vi "Read Test Parameters.vi"(8 "error in":errorcluster) -> (0 "error out":errorcluster, 1 "fbf_2 Pass Criteria":i32=3, 2 "fbf_1 Pass Criteria":i32=10, 3 "Array of tests":T1[](array[typedef]) {"Measurement Res." format="%.0f MHz"; "Blocking Signal" format="%#_gdBm"; "Wanted Signal" format="%#_gdBm"; "Upper Frequency" format="%.0f MHz"; "Lower Frequency" format="%.0f MHz"})   [LabVIEW 2013]
uses:
  Master Test Parameters.ctl
  <vilib>/Utility/config.llb/Config Data RefNum.ctl
  Globals/Blocking Performance Test Application Globals.vi
  <vilib>/Utility/config.llb/Read Key (Double).vi
  Globals/Test Criteria Global.vi
  <vilib>/Utility/config.llb/Read Key (U32).vi
  <vilib>/Utility/config.llb/Read Key (I32).vi
  <vilib>/Utility/config.llb/NI_LVConfig.lvlib
panel:
  out "Sections":i32
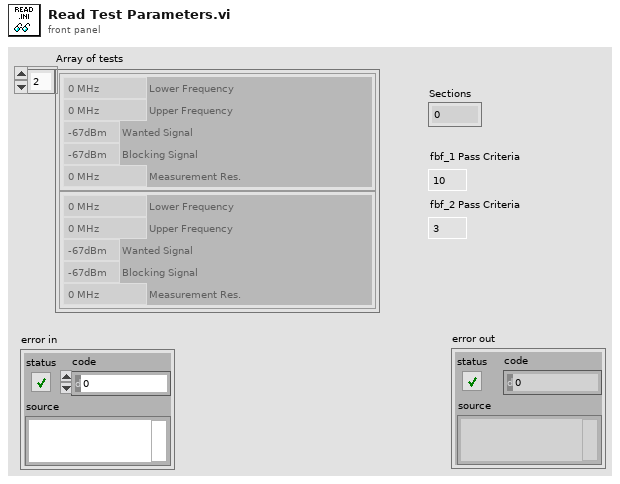
[diagram p1: front panel]
types:
  T1 = typedef "Master Test Parameters.ctl" = cluster{"Lower Frequency":u32, "Upper Frequency":u32, "Wanted Signal":dbl, "Blocking Signal":dbl, "Measurement Res.":u32}
  T2 = typedef "NI_LVConfig.lvlib/Config Data RefNum.ctl" = refnum<k1>
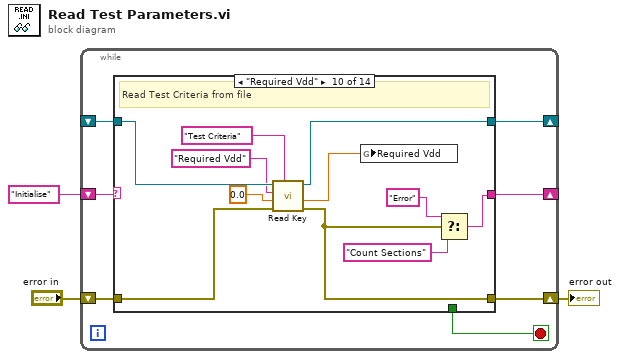
[diagram p0: block diagram]
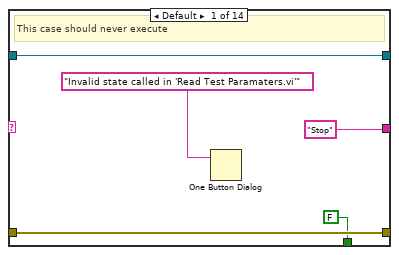
[diagram p2: hidden frame]
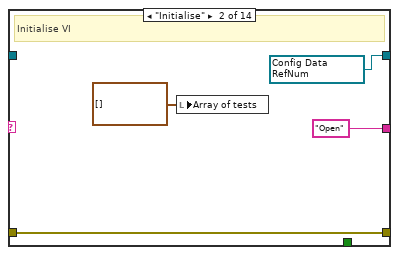
[diagram p3: hidden frame]
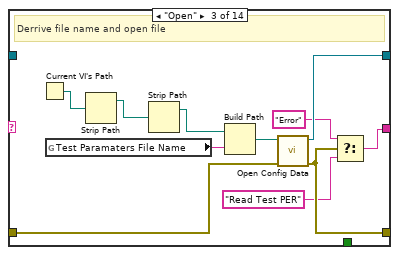
[diagram p4: hidden frame]
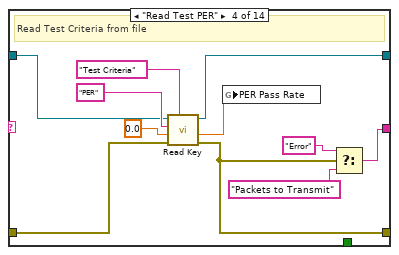
[diagram p5: hidden frame]
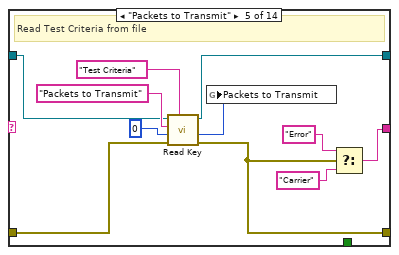
[diagram p6: hidden frame]
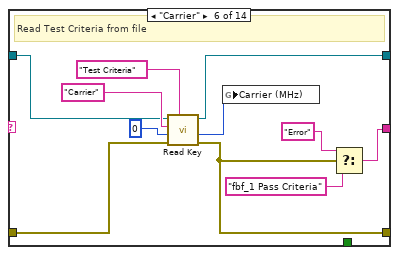
[diagram p7: hidden frame]
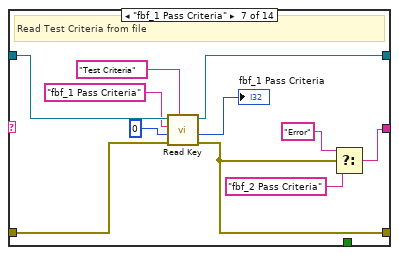
[diagram p8: hidden frame]
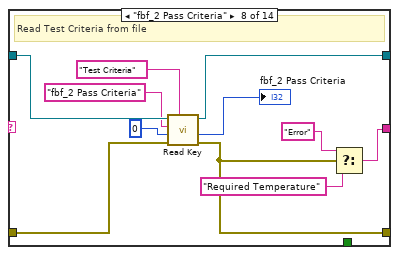
[diagram p9: hidden frame]
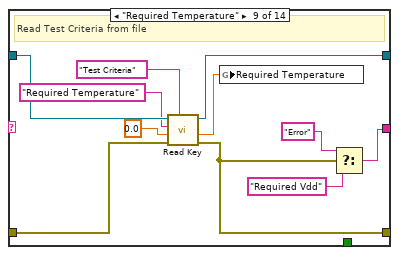
[diagram p10: hidden frame]
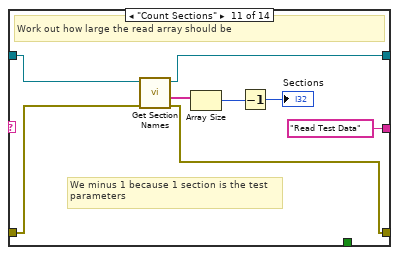
[diagram p11: hidden frame]
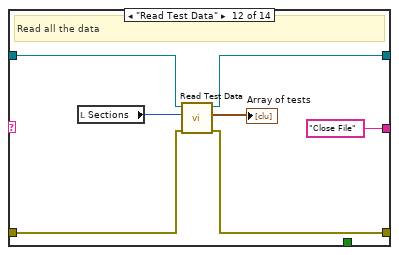
[diagram p12: hidden frame]
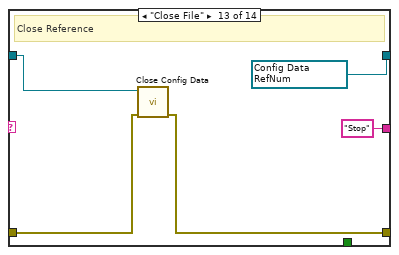
[diagram p13: hidden frame]
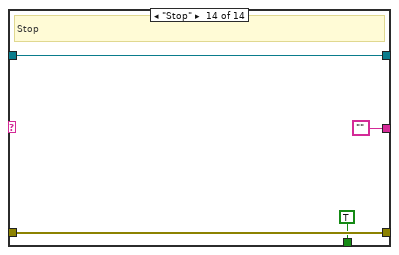
[diagram p14: hidden frame]
diagram:
  n1 = while {
    shift-right: [w9] -> _
    shift-left: "Initialise" -> [w10]
    shift-right: [w8] -> _
    shift-left: _ -> [w7]
    shift-right: [w6] -> w1
    shift-left: "error in" -> [w5]
    stop <- w4 stop-if-true
    n2 = case shown="\"Required Vdd\"" w10 {
      tunnel: ["Stop" "Open" w25 w35 w47 w57 w70 w81 w92 w103 "Read Test Data" ("section") "Close File" "Stop" ("section") ""] -> w9
      tunnel: [w15 w17 w24 w33 w44 w55 w68 w79 w90 w101 w114 w120 w126 w129] -> w8
      tunnel: w7 -> [w15 _ _ w34 w45 w56 w69 w80 w91 w102 w115 w121 w127 w129]
      tunnel: w5 -> [w12 w16 w23 w37 w49 w59 w72 w83 w94 w105 w110 w119 w125 w131]
      tunnel: [w12 w16 w22 w36 w48 w58 w71 w82 w93 w104 w109 w118 w124 w131] -> w6
      tunnel: [FALSE _ _ _ _ _ _ _ _ _ _ _ _ TRUE] -> w4
      frame Default {
        # "This case should never execute"
        n3 = One Button Dialog(message="Invalid state called in 'Read Test Paramaters.vi'") -> ()  [unwired: 1 in, 1 out]
      }
      frame "Initialise" {
        w17 = T2 refnum items=["config data"] ("refnum")
        # "Initialise VI"
        n4 = local write "Array of tests"(T1[] [] ("Array of tests")) -> ()
      }
      frame "Open" {
        # "Derrive file name and open file"
        n5 = Current VI's Path() -> (path=w27:path)
        n6 = global read "Blocking Performance Test Application Globals.vi" "Test Paramaters File Name"() -> (w28:string)
        n7 = Strip Path(path=w27) -> (stripped path=w29:path)  [unwired: 1 out]
        n8 = Strip Path(path=w29) -> (stripped path=w30:path)  [unwired: 1 out]
        n9 = Build Path(base path=w30, name or relative path=w28) -> (appended path=w26:path)
        n10 = call <vilib>:"Open Config Data.vi"("error in (no error)"=w23, "configuration file path"=w26) -> ("error out"=w22:errorcluster, "refnum"=w24:T2)  [unwired: 7 in, 1 out]
        n11 = Select(t="Error", s=w22, f="Read Test PER") -> (s? t:f=w25:string)
      }
      frame "Read Test PER" {
        # "Read Test Criteria from file"
        n12 = call-poly <vilib>:"Read Key.vi"("section"="Test Criteria", "error in (no error)"=w37, "default value"=0.0 ("PER Pass Rate"), "key"="PER", "refnum"=w34) -> ("error out"=w36:errorcluster, "value"=w41:dbl, "refnum out"=w33:T2)  [unwired: 3 in, 1 out]
        n13 = global write "Test Criteria Global.vi" "PER Pass Rate"(w41) -> ()
        n14 = Select(t="Error" ("section"), s=w36, f="Packets to Transmit" ("section")) -> (s? t:f=w35:string)
      }
      frame "Packets to Transmit" {
        # "Read Test Criteria from file"
        n15 = call-poly <vilib>:"Read Key.vi"("section"="Test Criteria", "error in (no error)"=w49, "default value"=u32 0 ("PER Pass Rate"), "key"="Packets to Transmit", "refnum"=w45) -> ("error out"=w48:errorcluster, "value"=w52:u32, "refnum out"=w44:T2)  [unwired: 3 in, 1 out]
        n16 = global write "Test Criteria Global.vi" "Packets to Transmit"(w52) -> ()
        n17 = Select(t="Error" ("section"), s=w48, f="Carrier" ("section")) -> (s? t:f=w47:string)
      }
      frame "Carrier" {
        # "Read Test Criteria from file"
        n18 = call-poly <vilib>:"Read Key.vi"("section"="Test Criteria", "error in (no error)"=w59, "default value"=u32 0 ("PER Pass Rate"), "key"="Carrier", "refnum"=w56) -> ("error out"=w58:errorcluster, "value"=w63:u32, "refnum out"=w55:T2)  [unwired: 3 in, 1 out]
        n19 = global write "Test Criteria Global.vi" "Carrier (MHz)"(w63) -> ()
        n20 = Select(t="Error" ("section"), s=w58, f="fbf_1 Pass Criteria" ("section")) -> (s? t:f=w57:string)
      }
      frame "fbf_1 Pass Criteria" {
        # "Read Test Criteria from file"
        n21 = call-poly <vilib>:"Read Key.vi"("section"="Test Criteria", "error in (no error)"=w72, "default value"=0 ("PER Pass Rate"), "key"="fbf_1 Pass Criteria", "refnum"=w69) -> ("error out"=w71:errorcluster, "value"=→"fbf_1 Pass Criteria":i32, "refnum out"=w68:T2)  [unwired: 3 in, 1 out]
        n22 = Select(t="Error" ("section"), s=w71, f="fbf_2 Pass Criteria" ("section")) -> (s? t:f=w70:string)
      }
      frame "fbf_2 Pass Criteria" {
        # "Read Test Criteria from file"
        n23 = call-poly <vilib>:"Read Key.vi"("section"="Test Criteria", "error in (no error)"=w83, "default value"=0 ("PER Pass Rate"), "key"="fbf_2 Pass Criteria", "refnum"=w80) -> ("error out"=w82:errorcluster, "value"=→"fbf_2 Pass Criteria":i32, "refnum out"=w79:T2)  [unwired: 3 in, 1 out]
        n24 = Select(t="Error" ("section"), s=w82, f="Required Temperature" ("section")) -> (s? t:f=w81:string)
      }
      frame "Required Temperature" {
        # "Read Test Criteria from file"
        n25 = call-poly <vilib>:"Read Key.vi"("section"="Test Criteria", "error in (no error)"=w94, "default value"=0.0 ("PER Pass Rate"), "key"="Required Temperature", "refnum"=w91) -> ("error out"=w93:errorcluster, "value"=w86:dbl, "refnum out"=w90:T2)  [unwired: 3 in, 1 out]
        n26 = global write "Test Criteria Global.vi" "Required Temperature"(w86) -> ()
        n27 = Select(t="Error" ("section"), s=w93, f="Required Vdd" ("section")) -> (s? t:f=w92:string)
      }
      frame "Required Vdd" {
        # "Read Test Criteria from file"
        n28 = call-poly <vilib>:"Read Key.vi"("section"="Test Criteria", "error in (no error)"=w105, "default value"=0.0 ("PER Pass Rate"), "key"="Required Vdd", "refnum"=w102) -> ("error out"=w104:errorcluster, "value"=w97:dbl, "refnum out"=w101:T2)  [unwired: 3 in, 1 out]
        n29 = global write "Test Criteria Global.vi" "Required Vdd"(w97) -> ()
        n30 = Select(t="Error" ("section"), s=w104, f="Count Sections" ("section")) -> (s? t:f=w103:string)
      }
      frame "Count Sections" {
        # "We minus 1 because 1 section is the test\nparameters"
        # "Work out how large the read array should be"
        n31 = call <vilib>:"Get Section Names.vi"("error in (no error)"=w110, "refnum"=w115) -> ("error out"=w109:errorcluster, "section names"=w113:string[], "refnum out"=w114:T2)  [unwired: 7 in]
        n32 = Array Size(array=w113) -> (size(s)=w112:i32)
        n33 = Decrement(x=w112) -> (x-1=→"Sections":i32)
      }
      frame "Read Test Data" {
        # "Read all the data"
        n34 = local read "Sections"() -> (w122:i32)
        n35 = call "Read Test Data.vi"("error in"=w119, "Sections"=w122, "refnum"=w121) -> ("error out"=w118:errorcluster, "Array of tests"=→"Array of tests":T1[], "refnum out"=w120:T2)  [unwired: 6 in]
      }
      frame "Close File" {
        w126 = T2 refnum items=["config data"] ("refnum out")
        # "Close Reference"
        n36 = call <vilib>:"Close Config Data.vi"("error in (no error)"=w125, "refnum"=w127) -> ("error out"=w124:errorcluster)  [unwired: 8 in, 1 out]
      }
      frame "Stop" {
        # "Stop"
      }
    }
  }
  "error out" <- w1
